vi "Actor Core.vi"(8 "error in":errorcluster caption="错误输入", 11 "MainPage in":refnum<class "MainPage.lvclass"> caption="操作者输入") -> (0 "error out":errorcluster caption="错误输出", 3 "Actor out":refnum<class "Actor.lvclass"> caption="操作者输出")   [LabVIEW 2019, in "MainPage.lvlib" / "MainPage.lvclass"]
doc: "(<B>文件名</B>: Actor Framework.lvlib:Actor.lvclass:Actor Core.vi)\n\n接收发送至操作者的消息，响应消息并处理可能导致操作者关闭的错误。\n\n子孙类重写该VI，使操作者完成特定的任务。使用调用父方法节点实现重写。"
uses:
  MainPage.lvclass
  D:/Program Files (x86)/National Instruments/LabVIEW 2019/vi.lib/ActorFramework/Actor/Actor.lvclass
  <vilib>/ActorFramework/Actor/Actor.lvclass
  <vilib>/ActorFramework/Actor/Actor.lvclass/Actor.ctl
  <vilib>/ActorFramework/Message Enqueuer/Message Enqueuer.lvclass/Message Enqueuer.ctl
  MainPage.lvclass/MainPage.ctl
  d72534ae-1d72-4a8f-8c68-5dbac9a72bc5.vi
  c7a1116b-e9b1-4e5e-808a-6794f7e89e26.vi
  4dc50e0b-562a-4a7b-a092-2ff577ba7486.vi
  84c122f6-6e4f-4dc9-8153-010595f57639.vi
  af074030-de50-4ce2-9988-cab0e81f1129.vi
  83de82aa-53b3-4bbc-a1df-207bde8d7e65.vi
  c0120f8a-0871-459c-b341-a9ac3cf3e51c.vi
  <vilib>/numeric/Random Number (Range) U64.vi
  <vilib>/ActorFramework/Message Enqueuer/Init from Existing Queue.vi
  <vilib>/ActorFramework/Message Enqueuer/Enqueue.vi
  <vilib>/numeric/sub_Random U32.vi
  <vilib>/ActorFramework/Stop Msg/Stop Msg.lvclass
  D:/Program Files (x86)/National Instruments/LabVIEW 2019/vi.lib/ActorFramework/Message/Message.lvclass
  <vilib>/ActorFramework/Message Priority Queue/Priority Enqueue.vi
  <vilib>/ActorFramework/Message Enqueuer/Message Enqueuer.lvclass
panel:
  in  "动作设置":T1={"模拟寄存器重置"=enum."址值一致", "值"=0, "数量"=1500, "CRC计算"=FALSE}
  in  "停止按钮":bool
  in  "报文解析显示界面":enum32{"选项卡 1", "选项卡 2", "选项卡 3", "选项卡 4"}(tab)
  in  "03去重":bool=TRUE caption="03指令去重？"
  out "报文流水显示":string
  out "错误报文":string[][](table) caption="MB RTU 解析失败报文"
  out "03":string[][](table) caption="功能码 03"
  out "06":string[][](table) caption="功能码 06"
  out "16":string[][](table) caption="功能码 16（0X10）"
  in  "命令发送":bool
  in  "发送输入":string
  in  "清除记录":bool
  in  "连接断开":bool
  in  "连接启用":bool
  in  "寄存器重置":bool
  in  "界面选择":enum32{"界面 1", "界面 2", "界面 3", "界面 4"}(radio)
  in  "配置选择":enum32{"串口连接", "服务端", "客服端"}(tab)
  in  "串口配置":T2={"VISA串口名称"="", "波特率"=9600, "停止位"=10, "流控制"=0, "数据位"=8, "奇偶校验"=enum."None", "超时"=2000, "启用终止符？"=FALSE, "终止符"=10} {"终止符" format="%.0x"; "数据位" min=5 max=8 step=1; "流控制" items=["无", "XON/XOFF", "RTS/CTS", "XON/XOFF & RTS/CTS", "DTR/DSR", "XON/XOFF & DTR/DSR"]; "停止位" items=["1.0"=10, "1.5"=15, "2.0"=20]; "波特率" items=["9600"=9600, "115200"=15]}
  in  "服务端配置":cluster{"本机 IP":string, "侦听端口":u16}={"本机 IP"="", "侦听端口"=4001}
  in  "服务端选择":cluster{"设备选择":string}
  in  "客服端配置":T3={"本机 IP\n(仅供浏览)"="", "本机端口"=5001, "主机 IP"="127.0.0.1", "主机端口"=4001}
  in  "客服端选择":cluster{"客P-主IP:Port":string}
  out "状态条":T4
  in  "通用配置":T5={"ModBusRTU反馈"=enum."无反馈", "侦听周期"=0, "跳转反馈"=FALSE, "报文记录数量"=0, "客服端新增模式"=enum."单端模式"}
  out "模拟寄存器":u16[](array[numeric])
  # "后续更新：\n后边增加监听模式\n即侦听主从通讯信息，分析两方报文"
  # "常规设置增加反馈延时？？\n测试反馈不及时的时间？？"
  # "未实装\n    ↓"
  # "侦听周期是等待时间\n触发侦听是 首次侦听设置+10ms 时间触发一次侦听\n所以这里存在问题，后续时间只能小，不能大"
  # "地址"
  # "+0"
  # "+5"
  # "+10"
  # "错误反馈配置\n\n更改对应的属性\n  如 通讯地址 功能码  寄存器地址  等\n是否计算crc16 ，及 正确？"
  # "初始化是1500-址值一致"
  # "命令设置"
  # "ModbusRTU\n内置解析范围，当前针对功能码：03 06 16(十进制数)\n接收只针对询问报文的拆解，其它类型会被划分为未知命令\n\n示例格式(00代表U8字符，0000即U16字符，十六进制字符串显示)\n03询问：    01          03        0000         0001        XXXX \n            通讯地址  功能码  寄存器地址  需求数据量  CRC16\n03反馈：    01          03          00           0000 ... 0000         XXXX \n            通讯地址  功能码  数据字节量  数据段(根据询问反馈)  CRC16\n    **字节量代表U8数量，是数据量（U16字）的两倍。\n06下发/反馈  一致\n                01         06          0000      0000    XXXX\n            通讯地址  功能码  寄存器地址  写入值  CRC16\n16下发\n               01           10        0000        0001        02        0000     XXXX\n            通讯地址  功能码  寄存器地址  数据量  数据字节量  数据段  CRC16 \n16反馈\n               01          10        0000       0001    XXXX\n           通讯地址  功能码  寄存器地址  数据量  CRC16\n\n接收报文解析，只针对于询问/下发做拆解反馈"
  # "目前已完成功能：\n  1.串口和TCP两模式，共3种情况的连接。及切换逻辑\n      同一时间只能存在一种连接方式。不能并存。虽然可以达成并存实现。\n  2.模拟设备，接收询问/下发指令并拆解分类显示\n    模拟设备，根据报文反馈/修改 模拟寄存器的值。\n    **用于常见的命令接收测试，方便直观查看命令数据情况\n    ***不准备集成通讯协议(没有必要，而且通讯协议输入存在问题可能会导致错误判断)\n    ***错误反馈拓展当前未想好怎么做，已预留接口\n\n\n正在进行中：\n  1.错误反馈设置及实装\n  2.主动通讯模式设置及实装（原有模式存在时间控制问题）\n  3.主动通讯配置/功能的明确及实现\n  4."
  # "后续拓展功能：（预期）\n监听模式：即充当第三方监听通讯的收发报文，并能处理识别分类报文\n侦听反馈延时：侦听报文后，增加延迟回复。某些情况下测试极限反应时间\n\n\n\n\n需要更改/更新/修正/bug\n1.侦听等待，侦听触发周期，拓展发收模式的时间控制。比较混乱需要重新考虑，是否增加参数。防止时间冲突导致堵塞之类的情况\n2.配置，信息记录，数据记录独立分散。不太好管理处理，调用过多。考虑怎么处理好一些。看看是否方便修改\n3.某些读取VI，调用太过频繁和耗时。需要性能整改\n\n4.**无法解决**在服务端和客服端通讯的情况下，两端无实际通讯的情况注销连接，服务端无法重新侦听显示端口占用。涉及TCP通讯，目前没有头绪。\n\n5.**无法解决**本电脑第一次扫描端口（串口）会卡大半天。初步判断和电脑有关。"
  # "实际+10ms间隔时间"
  # "达到上限会顶替旧记录"
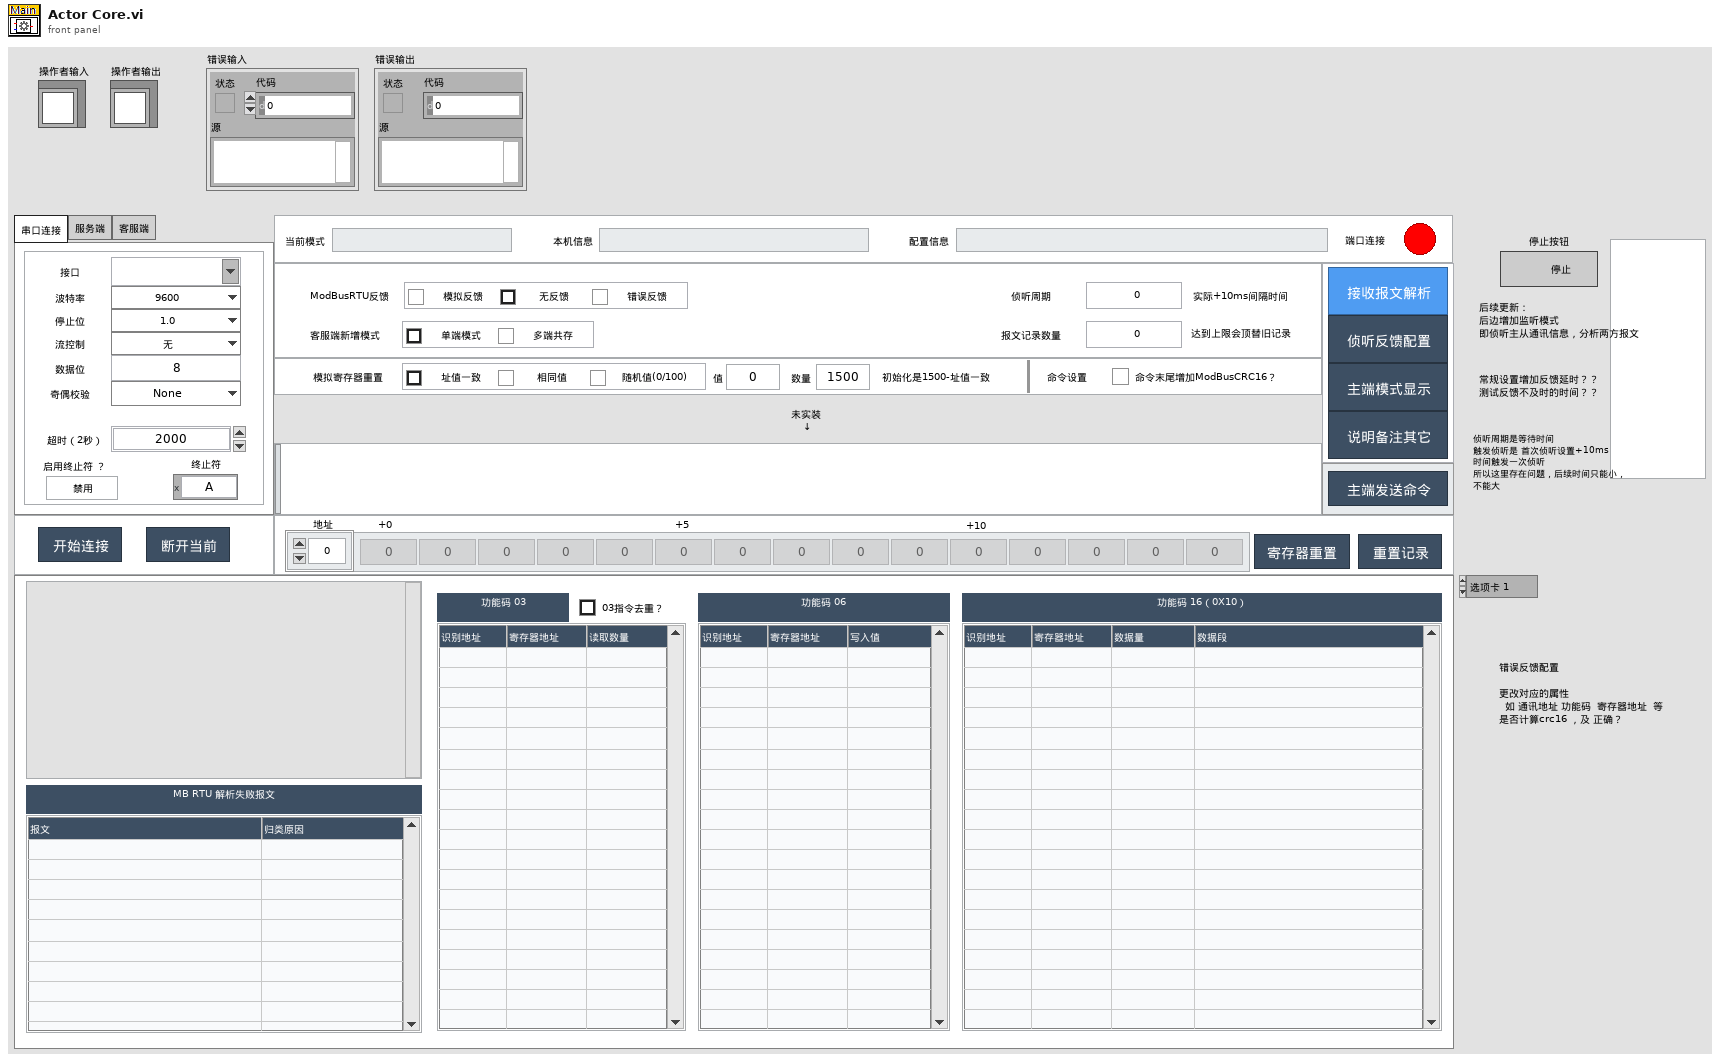
[diagram p1: front panel]
types:
  T1 = cluster{"模拟寄存器重置":enum32{"址值一致", "相同值", "随机值(0/100)"}, "值":u16, "数量":u16, "CRC计算":bool}
  T2 = cluster{"VISA串口名称":refnum<visa-resource-name>, "波特率":u32, "停止位":u16, "流控制":u16, "数据位":u16, "奇偶校验":enum16{"None", "Odd", "Even", "Mark", "Space"}, "超时":u32, "启用终止符？":bool, "终止符":u8}
  T3 = cluster{"本机 IP\n(仅供浏览)":string, "本机端口":u16, "主机 IP":string, "主机端口":u16}
  T4 = cluster{"当前模式":string, "本机信息":string, "配置信息":string, "端口连接":bool}
  T5 = typedef "MainPage.lvlib/MainPage.lvclass/通用配置选项.ctl" = cluster{"ModBusRTU反馈":enum32{"模拟反馈", "无反馈", "错误反馈"}, "侦听周期":u32, "跳转反馈":bool, "报文记录数量":u16, "客服端新增模式":enum32{"单端模式", "多端共存"}}
  T6 = cluster{"寄存器模拟":u16[], "串口正常？":bool, "报文信息记录":string[][]}
  T7 = enum16{"ini", "增加记录", "读取记录", "更改寄存器值", "更改接口状态", "更改报文信息", "增加报文信息"}
  T8 = cluster{"串口正常？":bool, "寄存器模拟":u16[], "报文信息记录":string[][]}
  T9 = enum16{"ini", "读取", "写入-报文记录", "写入-寄存器模拟", "写入-串口状态", "增加报文记录"}
  T10 = typedef "MainPage.lvlib/MainPage.lvclass/DataRef_通讯接口.ctl" = cluster{"连接方式":enum16{"网口(客服端)", "网口(服务端)", "串口"}, "VISA串口名称":refnum<visa-resource-name>, "服务端识别":cluster{"本机IP":string, "本机端口":u16, "当前目标":string}, "客服端识别":cluster{"客P-主IP:Port":string}, "服务端记录":cluster{"服务端侦听ID":refnum<k5>, "服务端接口记录":map{string, refnum<k5>}}, "客服端记录":map{string, refnum<k5>}}
  T11 = enum32{"Invalid", "Standard", "Closed", "Hidden", "Minimized", "Maximized"}
  T12 = cluster{"模式":string, "本机信息":string, "目标信息":string, "串口正常？":bool}
  T13 = cluster{"报文":string, "类别":string, "拆分属性":cluster{"通讯地址":string, "功能码":string, "寄存器地址":string, "数据":string, "16数据量":string}, "备注":string}[]
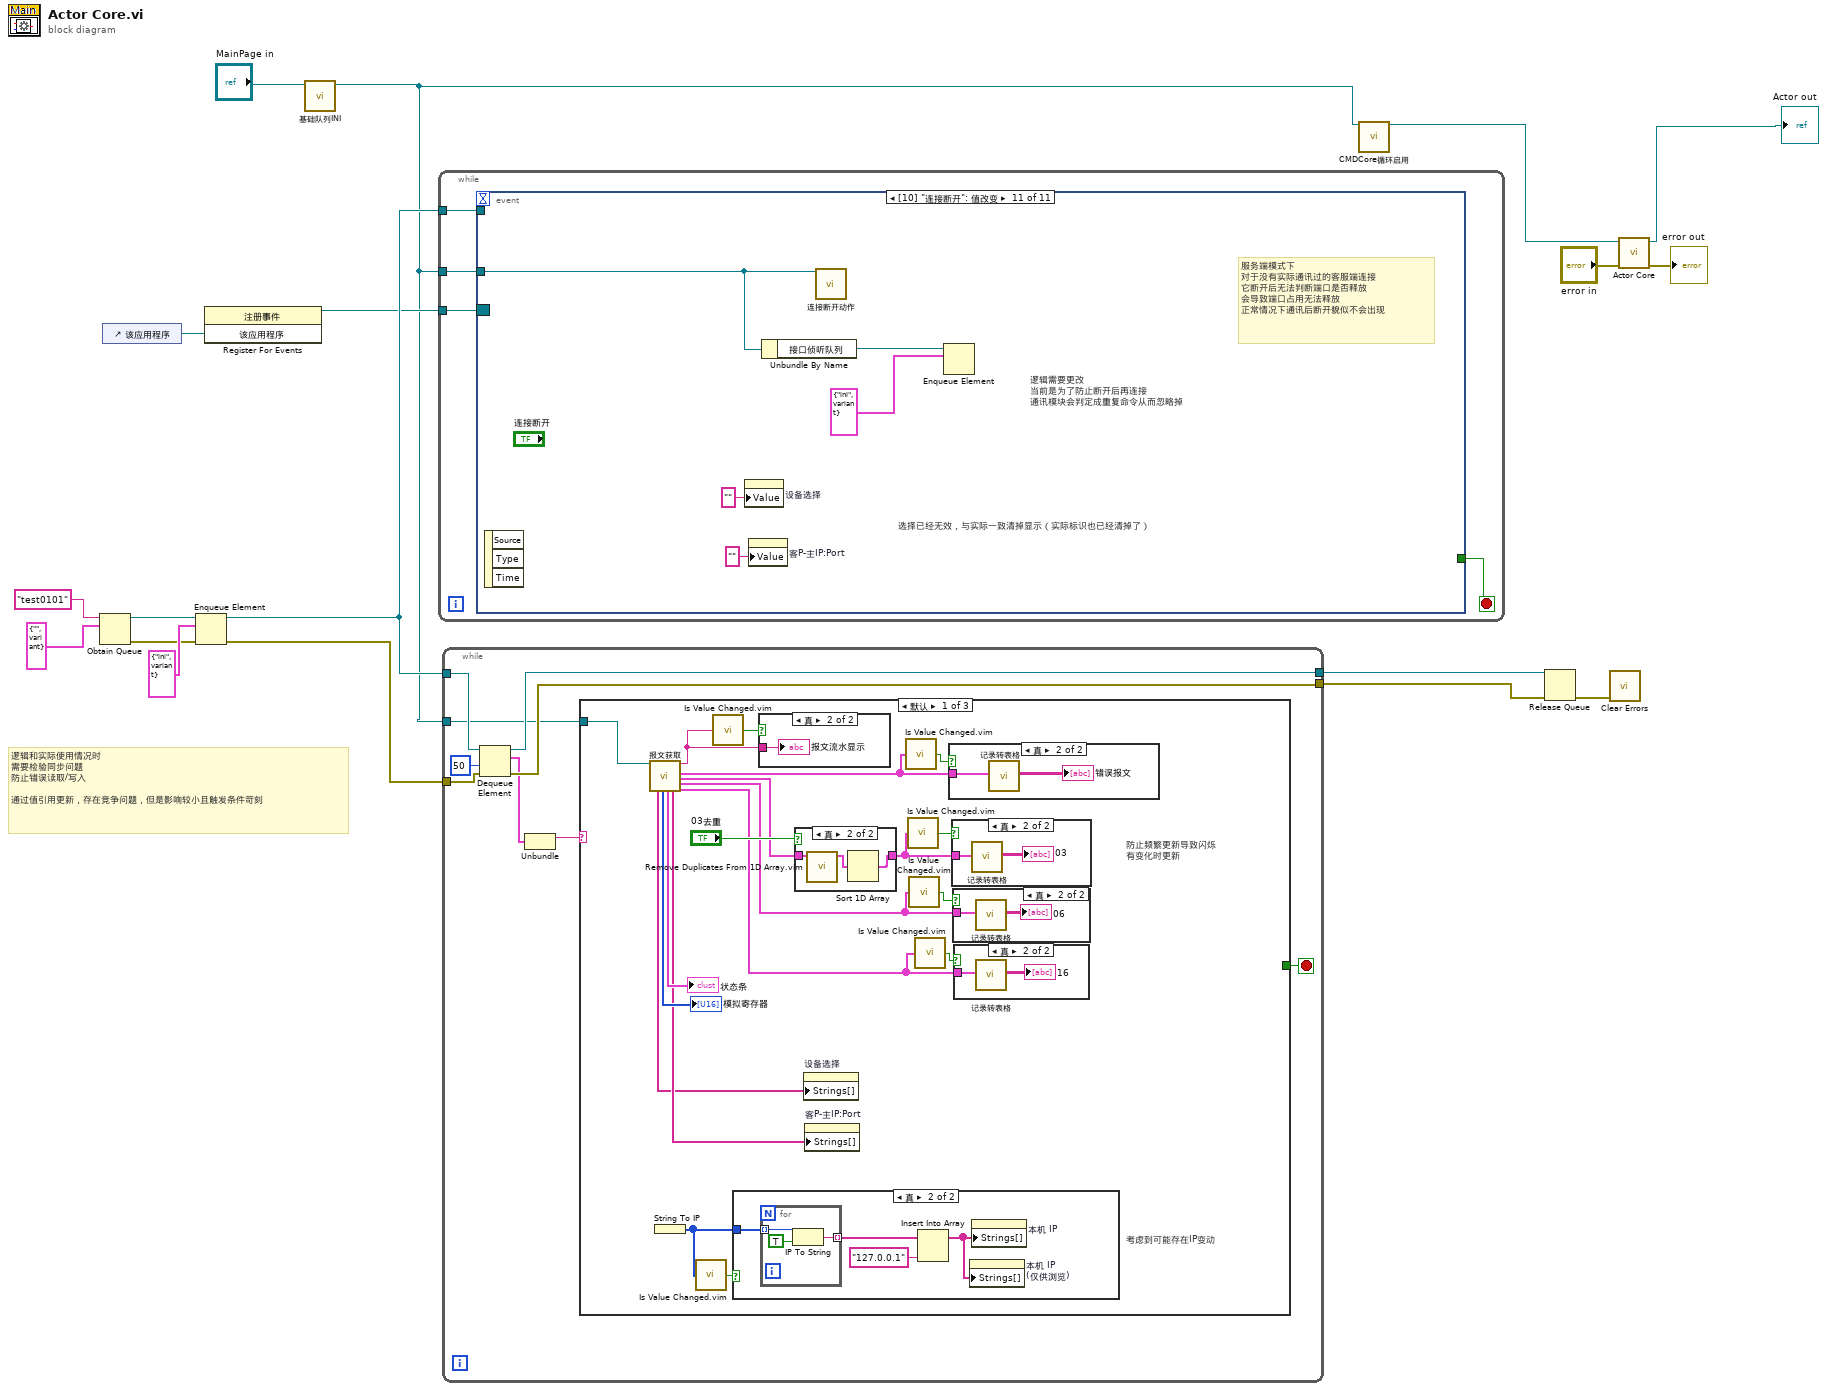
[diagram p0: block diagram]
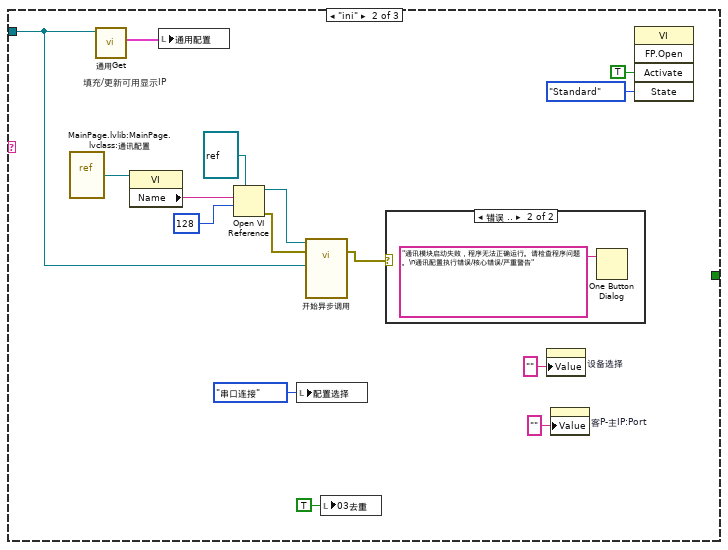
[diagram p9: hidden frame]
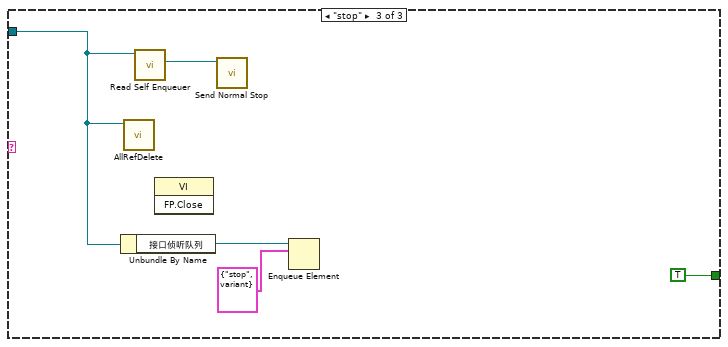
[diagram p11: hidden frame]
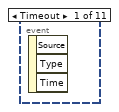
[diagram p12: hidden frame]
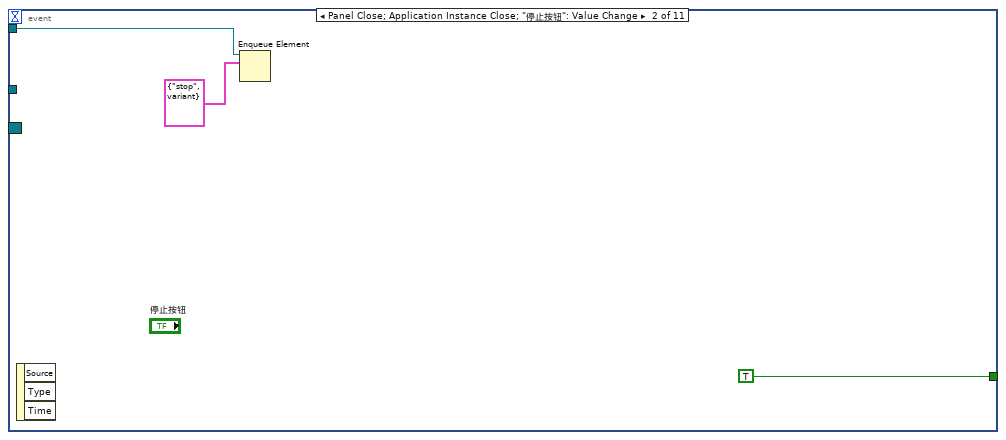
[diagram p13: hidden frame]
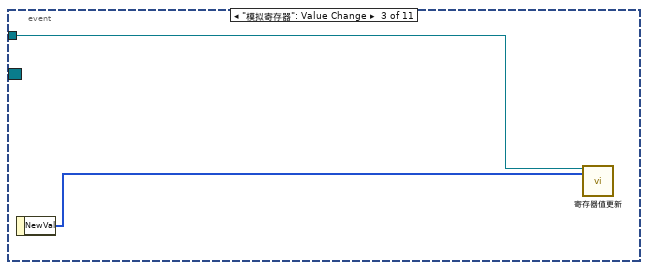
[diagram p14: hidden frame]
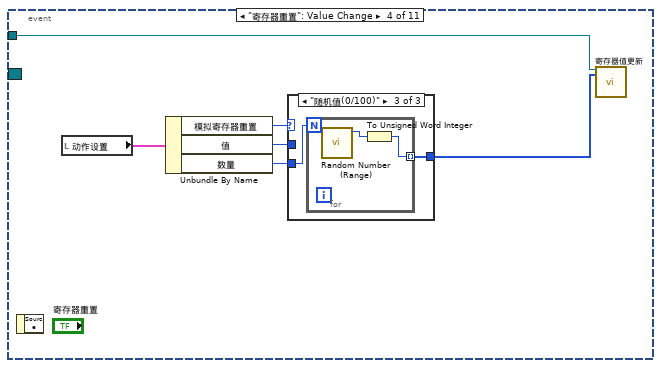
[diagram p15: hidden frame]
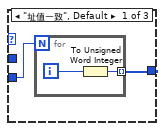
[diagram p16: hidden frame]
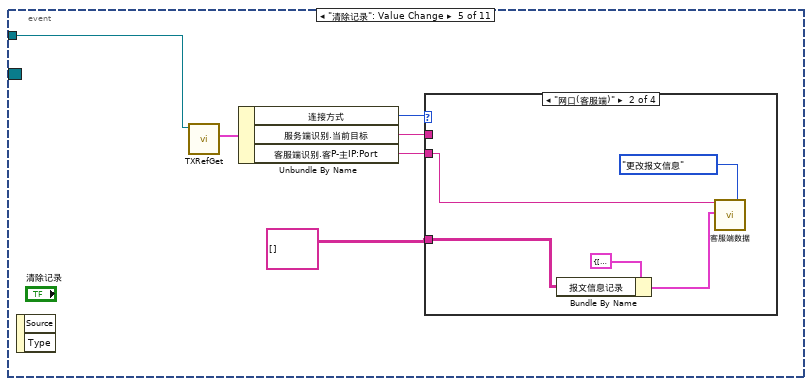
[diagram p18: hidden frame]
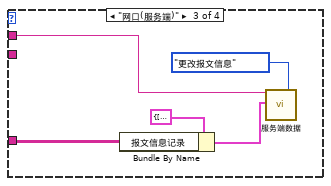
[diagram p20: hidden frame]
diagram:
  # "逻辑和实际使用情况时\n需要检验同步问题\n防止错误读取/写入\n\n通过值引用更新，存在竞争问题，但是影响较小且触发条件苛刻"
  n1 = Obtain Queue(name (unnamed)="test0101" ("名称（未命名）"), element data type=cluster{string, variant} {"", variant}) -> (queue out=w14:refnum<queue>, error out=w12:errorcluster)  [unwired: 3 in, 1 out]
  n2 = control-ref of="该应用程序"() -> (w6:refnum<vi>)
  n3 = Enqueue Element(queue=w14, element=cluster{string, variant} {"ini", variant} ("元素"), error in (no error)=w12) -> (queue out=w11:refnum<queue>, error out=w10:errorcluster)  [unwired: 1 in, 1 out]
  n4 = register-events(w6) -> (reference out=w5:refnum<event-registration>)  [unwired: 2 in, 1 out]
  n5 = call-dynamic "基础队列INI.vi"("MainPage 输入"="MainPage in") -> ("MainPage 输出"=w2:refnum<class "MainPage.lvclass">)  [unwired: 9 in, 1 out]
  n6 = while {
    tunnel: w11 -> [w22]
    tunnel: w2 -> [w21]
    tunnel: w5 -> [w19]
    stop <- w20 stop-if-true
    n7 = event shown="[10] \"连接断开\": 值改变" {
      selector: w19 -> [_ _ _ _ _ _ _ _ _ _ _]
      dyn-events: _ -> [_ _ _ _ _ _ _ _ _ _ _]
      timeout: _ -> [_ _ _ _ _ _ _ _ _ _ _]
      tunnel: w22 -> [_ w24 _ _ _ _ _ _ _ _ _]
      tunnel: w21 -> [_ _ w27 w29 w47 w66 w79 _ w93 w97 w121]
      tunnel: [_ TRUE ("停止按钮") _ _ _ _ _ _ _ _ _] -> w20
      event Timeout {
        n8 = event-data() -> ()  [unwired: 1 in, 3 out]
      }
      event Panel Close; Application Instance Close; "停止按钮": Value Change {
        n9 = event-data() -> ()  [unwired: 1 in, 3 out]
        n10 = Enqueue Element(queue=w24, element=cluster{string, variant} {"stop", variant} ("元素")) -> ()  [unwired: 2 in, 3 out]
      }
      event "模拟寄存器": Value Change {
        n11 = event-data() -> ("NewVal"=w26:u16[])  [unwired: 1 in]
        n12 = call "寄存器值更新.vi"("MainPage输入"=w27, "NewVal"=w26) -> ()  [unwired: 18 in]
      }
      event "寄存器重置": Value Change {
        n13 = event-data() -> ()  [unwired: 1 in, 1 out]
        n14 = local read "动作设置"() -> (w33:T1)
        n15 = Unbundle By Name(w33) -> ("模拟寄存器重置"=w32:enum32{"址值一致", "相同值", "随机值(0/100)"}, "值"=w31:u16, "数量"=w30:u16)
        n16 = case shown="\"随机值(0/100)\"" w32 {
          tunnel: w31 -> [_ w39 _]
          tunnel: w30 -> [w35 w38 w43]
          tunnel: [w34 w40 w42] -> w28
          frame "址值一致", Default {
            n17 = for {
              N: w35 -> [_]
              tunnel: [w36] -> w34 mode=indexing
              i -> [w37]
              n18 = To Unsigned Word Integer(number=w37) -> (unsigned 16bit integer=w36:u16)
            }
          }
          frame "相同值" {
            n19 = for {
              N: w38 -> [_]
              tunnel: [w41] -> w40 mode=indexing
              tunnel: w39 -> [w41]
            }
          }
          frame "随机值(0/100)" {
            n20 = for {
              N: w43 -> [_]
              tunnel: [w44] -> w42 mode=indexing
              n21 = call-poly <vilib>:"Random Number (Range).vi"() -> ("number"=w45:u64)  [unwired: 11 in]
              n22 = To Unsigned Word Integer(number=w45) -> (unsigned 16bit integer=w44:u16)
            }
          }
        }
        n23 = call "寄存器值更新.vi"("MainPage输入"=w29, "NewVal"=w28) -> ()  [unwired: 18 in]
      }
      event "清除记录": Value Change {
        n24 = event-data() -> ()  [unwired: 1 in, 2 out]
        n25 = call-dynamic "TXRefGet.vi"("MainPage 输入"=w47) -> ("通讯接口数据"=w48:T10)  [unwired: 6 in, 4 out]
        n26 = Unbundle By Name(w48) -> ("连接方式"=w51:enum16{"网口(客服端)", "网口(服务端)", "串口"}, "服务端识别.当前目标"=w49:string, "客服端识别.客P-主IP:Port"=w50:string)
        n27 = case shown="\"网口(客服端)\"" w51 {
          tunnel: w49 -> [_ _ w60 _]
          tunnel: w50 -> [_ w55 _ _]
          tunnel: string[][] [] ("报文信息记录") -> [_ w53 w58 w63]
          frame Default {
          }
          frame "网口(客服端)" {
            n28 = Bundle By Name(cluster=T6 {"寄存器模拟"=[], "串口正常？"=FALSE, "报文信息记录"=[]} ("数据输入"), "报文信息记录"=w53) -> (w52:T6)
            n29 = call "客服端数据.vi"("客P-主IP:P"=w55, "数据输入"=w52, "枚举"=T7."更改报文信息") -> ()  [unwired: 15 in, 2 out]
          }
          frame "网口(服务端)" {
            n30 = Bundle By Name(cluster=T6 {"寄存器模拟"=[], "串口正常？"=FALSE, "报文信息记录"=[]} ("数据输入"), "报文信息记录"=w58) -> (w57:T6)
            n31 = call "服务端数据.vi"("IP-Port"=w60, "数据输入"=w57, "枚举"=T7."更改报文信息") -> ()  [unwired: 15 in, 2 out]
          }
          frame "串口" {
            n32 = Bundle By Name(cluster=T8 {"串口正常？"=FALSE, "寄存器模拟"=[], "报文信息记录"=[]} ("串口输入"), "报文信息记录"=w63) -> (w62:T8)
            n33 = call "串口数据.vi"("串口输入"=w62, "枚举"=T9."写入-报文记录") -> ()  [unwired: 17 in, 1 out]
          }
        }
      }
      event "命令发送": Value Change {
        # "考虑使用队列传输记录\n逐步执行防止冲突"
        # "需要调取是否需要增加CRC的选项\n这里为了简单直接调取，而不是再次读取配置"
        n34 = event-data() -> ()  [unwired: 1 in, 2 out]
        n35 = Unbundle By Name("动作设置") -> ("CRC计算"=w68:bool)
        n36 = case shown="真" w68 {
          tunnel: "发送输入" -> [w70 w73]
          tunnel: [w70 w71] -> _
          frame False {
          }
          frame True {
            n37 = String To Byte Array(string=w73) -> (unsigned byte array=w72:u8[])
            n38 = call "CRC计算.vi"("无校验U8数组"=w72) -> ("计算后字符串"=w71:string)  [unwired: 17 in, 1 out]
          }
        }
        n39 = Unbundle By Name(w66) -> ()  [unwired: 1 out]
      }
      event "客服端选择.客P-主IP:Port", "服务端选择.设备选择": Value Change {
        # "同步，预期在模式切换时就可以直接适配读取\n但是存在逻辑上的问题\n模式切换时，会注销其它模式的连接，理论上，其它模式被重置后，是没有选择的。"
        n40 = event-data() -> ()  [unwired: 1 in, 1 out]
        n41 = call-dynamic "TXRefGet.vi"("MainPage 输入"=w79) -> ("引用"=w78:refnum<data-value>)  [unwired: 6 in, 4 out]
        n42 = Unbundle By Name("客服端选择") -> ("客P-主IP:Port"=w76:string)
        n43 = Unbundle By Name("服务端选择") -> ("设备选择"=w74:string)
        n44 = in-place {
          in-place-border: w76 -> [w82]
          in-place-border: w74 -> [w81]
          n45 = in-place-dvr #1(w78) -> (w83:T10)  [unwired: 1 out]
          n46 = Bundle By Name(cluster=w83, "服务端识别.当前目标"=w81, "客服端识别.客P-主IP:Port"=w82) -> (w80:T10)
          n47 = in-place-dvr #1(w80) -> ()  [unwired: 2 out]
        }
      }
      event "界面选择": Value Change {
        n48 = event-data() -> ()  [unwired: 1 in, 3 out]
        n49 = case shown="默认" "界面选择" {
          tunnel: [enum32{"选项卡 1", "选项卡 2", "选项卡 3", "选项卡 4"}."选项卡 1" ("报文解析显示界面") enum32{"选项卡 1", "选项卡 2", "选项卡 3", "选项卡 4"}."选项卡 1" ("报文解析显示界面") enum32{"选项卡 1", "选项卡 2", "选项卡 3", "选项卡 4"}."选项卡 2" ("报文解析显示界面") enum32{"选项卡 1", "选项卡 2", "选项卡 3", "选项卡 4"}."选项卡 3" ("报文解析显示界面") enum32{"选项卡 1", "选项卡 2", "选项卡 3", "选项卡 4"}."选项卡 4" ("报文解析显示界面")] -> w84
          frame Default {
          }
          frame "界面 1" {
          }
          frame "界面 2" {
          }
          frame "界面 3" {
          }
          frame "界面 4" {
          }
        }
        n50 = local write "报文解析显示界面"(w84) -> ()
      }
      event Value Change {
        n51 = event-data() -> ()  [unwired: 1 in, 1 out]
        n52 = call-dynamic "通用Get.vi"("MainPage 输入"=w93) -> ("通用引用"=w92:refnum<data-value>)  [unwired: 6 in, 4 out]
        n53 = in-place {
          in-place-border: "通用配置" -> [w94]
          n54 = in-place-dvr #2(w92) -> ()  [unwired: 2 out]
          n55 = in-place-dvr #2(w94) -> ()  [unwired: 2 out]
        }
      }
      event "连接启用": Value Change {
        n56 = event-data() -> ()  [unwired: 1 in, 3 out]
        n57 = Unbundle By Name(w97) -> ("接口侦听队列"=w95:refnum<queue>)
        n58 = case shown="\"客服端\"" "配置选择" {
          tunnel: w95 -> [_ w102 w108 w113]
          frame Default {
          }
          frame "串口连接" {
            n59 = To Variant(anything="串口配置") -> (Variant=w99:variant)
            n60 = Bundle("串口", "Variant"=w99) -> (w98:cluster{string, "Variant":variant})  [unwired: 1 in]
            n61 = Enqueue Element(queue=w102, element=w98) -> ()  [unwired: 2 in, 3 out]
          }
          frame "客服端" {
            n62 = Unbundle By Name("客服端配置") -> ("本机端口"=w106:u16, "主机 IP"=w105:string, "主机端口"=w104:u16)
            n63 = Bundle("本机端口"=w106, "主机 IP"=w105, "主机端口"=w104) -> (w103:cluster{"本机端口":u16, "主机 IP":string, "主机端口":u16})  [unwired: 1 in]
            n64 = To Variant(anything=w103) -> (Variant=w110:variant)
            n65 = Bundle("客服端", "Variant"=w110) -> (w109:cluster{string, "Variant":variant})  [unwired: 1 in]
            n66 = Enqueue Element(queue=w108, element=w109) -> ()  [unwired: 2 in, 3 out]
          }
          frame "服务端" {
            n67 = To Variant(anything="服务端配置") -> (Variant=w115:variant)
            n68 = Bundle("服务端", "Variant"=w115) -> (w114:cluster{string, "Variant":variant})  [unwired: 1 in]
            n69 = Enqueue Element(queue=w113, element=w114) -> ()  [unwired: 2 in, 3 out]
          }
        }
      }
      event "连接断开": Value Change {
        # "服务端模式下\n对于没有实际通讯过的客服端连接\n它断开后无法判断端口是否释放\n会导致端口占用无法释放\n正常情况下通讯后断开貌似不会出现"
        # "选择已经无效，与实际一致清掉显示（实际标识也已经清掉了）"
        # "逻辑需要更改\n当前是为了防止断开后再连接\n通讯模块会判定成重复命令从而忽略掉"
        n70 = event-data() -> ()  [unwired: 1 in, 3 out]
        n71 = property on="设备选择" class="CmbBox"("Value"="" ("值")) -> ()  [unwired: 2 in, 2 out]
        n72 = property on="客P-主IP:Port" class="CmbBox"("Value"="" ("值")) -> ()  [unwired: 2 in, 2 out]
        n73 = Unbundle By Name(w121) -> ("接口侦听队列"=w120:refnum<queue>)
        n74 = call "连接断开动作.vi"("MainPage 输入"=w121) -> ()  [unwired: 19 in]
        n75 = Enqueue Element(queue=w120, element=cluster{string, variant} {"ini", variant} ("元素")) -> ()  [unwired: 2 in, 3 out]
      }
    }
  }
  n76 = while {
    tunnel: w11 -> [w130]
    tunnel: [w128] -> w9
    tunnel: w10 -> [w127]
    tunnel: [w126] -> w8
    tunnel: w2 -> [w123]
    stop <- w122 stop-if-true
    n77 = Dequeue Element(queue=w130, timeout in ms (-1)=50 ("超时毫秒(-1)"), error in (no error)=w127) -> (queue out=w128:refnum<queue>, element=w125:cluster{string, variant}, error out=w126:errorcluster)  [unwired: 1 out]
    n78 = Unbundle(w125) -> (w124:string)  [unwired: 1 out]
    n79 = case shown="默认" w124 {
      tunnel: w123 -> [w149 w174 w188]
      tunnel: [_ _ TRUE] -> w122
      frame Default {
        # "考虑到可能存在IP变动"
        # "防止频繁更新导致闪烁\n有变化时更新"
        n80 = call "报文获取.vi"("MainPage"=w149) -> ("服务侦听设备"=w131:string[], "寄存器模拟"=→"模拟寄存器":u16[], "状态信息"=→"状态条":T12, "客服端-设备"=w132:string[], "流水显示"=w147:string, "未知记录"=w143:T13, "03记录"=w145:T13, "06记录"=w138:T13, "16记录"=w137:T13)  [unwired: 10 in]
        n81 = String To IP() -> (0:w134:u32[])  [unwired: 1 in]
        n82 = call "Is Value Changed.vim"("value"=w134) -> ("changed or first call?"=w133:bool)
        n83 = call "Is Value Changed.vim"("value"=w147) -> ("changed or first call?"=w148:bool)
        n84 = case shown="真" w133 {
          tunnel: w134 -> [_ w153]
          frame False {
          }
          frame True {
            n85 = for {
              tunnel: w153 -> [w155] mode=indexing
              tunnel: [w154] -> w152 mode=indexing
              n86 = IP To String(1:TRUE ("句点符号？(F)"), 2:w155) -> (0:w154:string)
            }
            n87 = Insert Into Array(array=w152, new element="127.0.0.1" ("名称")) -> (w150:string[])  [unwired: 1 in]
            n88 = property on="本机 IP\n(仅供浏览)" class="CmbBox"("Strings[]"=w150) -> ()  [unwired: 2 in, 2 out]
            n89 = property on="本机 IP" class="CmbBox"("Strings[]"=w150) -> ()  [unwired: 2 in, 2 out]
          }
        }
        n90 = case shown="真" w148 {
          tunnel: w147 -> [_ w169]
          frame False {
          }
          frame True {
            "报文流水显示" <- w169
          }
        }
        n91 = case shown="真" "03去重" {
          tunnel: w145 -> [w165 w168]
          tunnel: [w165 w167] -> w140
          frame False {
          }
          frame True {
            n92 = call "Remove Duplicates From 1D Array.vim"("array"=w168) -> ("array with duplicates removed"=w166:T13)  [unwired: 10 in]
            n93 = Sort 1D Array(array=w166) -> (sorted array=w167:T13)
          }
        }
        n94 = property on="设备选择" class="CmbBox"("Strings[]"=w131) -> ()  [unwired: 2 in, 2 out]
        n95 = property on="客P-主IP:Port" class="CmbBox"("Strings[]"=w132) -> ()  [unwired: 2 in, 2 out]
        n96 = call "Is Value Changed.vim"("value"=w143) -> ("changed or first call?"=w142:bool)
        n97 = call "Is Value Changed.vim"("value"=w140) -> ("changed or first call?"=w141:bool)
        n98 = call "Is Value Changed.vim"("value"=w138) -> ("changed or first call?"=w139:bool)
        n99 = call "Is Value Changed.vim"("value"=w137) -> ("changed or first call?"=w136:bool)
        n100 = case shown="真" w142 {
          tunnel: w143 -> [_ w163]
          frame False {
          }
          frame True {
            n101 = call "记录转表格.vi"("记录"=w163) -> ("表格"=→"错误报文":string[][])  [unwired: 18 in]
          }
        }
        n102 = case shown="真" w141 {
          tunnel: w140 -> [_ w161]
          frame False {
          }
          frame True {
            n103 = call "记录转表格.vi"("记录"=w161) -> ("表格"=→"03":string[][])  [unwired: 18 in]
          }
        }
        n104 = case shown="真" w139 {
          tunnel: w138 -> [_ w160]
          frame False {
          }
          frame True {
            n105 = call "记录转表格.vi"("记录"=w160) -> ("表格"=→"06":string[][])  [unwired: 18 in]
          }
        }
        n106 = case shown="真" w136 {
          tunnel: w137 -> [_ w158]
          frame False {
          }
          frame True {
            n107 = call "记录转表格.vi"("记录"=w158) -> ("表格"=→"16":string[][])  [unwired: 18 in]
          }
        }
      }
      frame "ini" {
        # "填充/更新可用显示IP"
        n108 = vi-ref "MainPage.lvlib:MainPage.lvclass:通讯配置.vi"() -> (w179:refnum<vi>)
        n109 = call-dynamic "通用Get.vi"("MainPage 输入"=w174) -> ("通用配置"=w184:T5)  [unwired: 6 in, 4 out]
        n110 = property class="VI"(reference=w179) -> ("Name"=w178:string)  [unwired: 1 in, 2 out]
        n111 = local write "通用配置"(w184) -> ()
        n112 = Open VI Reference(type specifier VI Refnum (for type only)=refnum<vi> refnum ("类型说明符VI引用句柄（仅用于类型）"), vi path=w178, options=128 ("选项")) -> (vi reference=w180:refnum<vi>, error out=w176:errorcluster)  [unwired: 3 in]
        n113 = local write "配置选择"(enum32{"串口连接", "服务端", "客服端"}."串口连接" ("配置选择")) -> ()
        n114 = call-by-ref "开始异步调用"(reference=w180, error in=w176, "MainPage 输入"=w174) -> (error out=w175:errorcluster)  [unwired: 10 in, 2 out]
        n115 = local write "03去重"(TRUE ("03去重")) -> ()
        n116 = case shown="错误 .." w175 {
          frame No Error {
          }
          frame Error {
            n117 = One Button Dialog(message="通讯模块启动失败，程序无法正确运行。请检查程序问题。\n通讯配置执行错误/核心错误/严重警告" ("消息")) -> ()  [unwired: 1 in, 1 out]
          }
        }
        n118 = property on="设备选择" class="CmbBox"("Value"="" ("值")) -> ()  [unwired: 2 in, 2 out]
        n119 = property on="客P-主IP:Port" class="CmbBox"("Value"="" ("值")) -> ()  [unwired: 2 in, 2 out]
        n120 = invoke class="VI" method="FP.Open"("Activate"=TRUE ("激活？"), "State"=T11."Standard" ("状态")) -> ()  [unwired: 3 in, 5 out]
      }
      frame "stop" {
        n121 = Unbundle By Name(w188) -> ("接口侦听队列"=w187:refnum<queue>)
        n122 = call-dynamic "AllRefDelete.vi"("MainPage 输入"=w188) -> ()  [unwired: 9 in, 2 out]
        n123 = call <vilib>:"Read Self Enqueuer.vi"("Actor"=w188) -> ("Self Enqueuer"=w189:refnum<class "Message Enqueuer.lvclass">)  [unwired: 10 in]
        n124 = invoke class="VI" method="FP.Close"() -> ()  [unwired: 3 in, 3 out]
        n125 = call <vilib>:"Send Normal Stop.vi"("Message Enqueuer"=w189) -> ()  [unwired: 10 in, 1 out]
        n126 = Enqueue Element(queue=w187, element=cluster{string, variant} {"stop", variant} ("元素")) -> ()  [unwired: 2 in, 3 out]
      }
    }
  }
  n127 = call "CMDCore循环启用.vi"("MainPage输入"=w2) -> ("MainPage输出"=w1:refnum<class "MainPage.lvclass">)  [unwired: 18 in]
  n128 = Release Queue(queue=w9, error in (no error)=w8) -> (error out=w7:errorcluster)  [unwired: 1 in, 2 out]
  n129 = call <vilib>:"Clear Errors.vi"("error in (no error)"=w7) -> ()  [unwired: 5 in, 2 out]
  n130 = call-parent "Actor Core.vi"("error in"="error in", "Actor in"=w1) -> ("error out"=→"error out":errorcluster, "Actor out"=→"Actor out":refnum<class "Actor.lvclass">)  [unwired: 8 in]
